vi "Empty Position.vi"(4 "Col":i32, 6 "Row":i32, 10 "Team In":i32[][](array[numeric]), 11 "Squares In":refnum<class "Square.lvclass">[][](array[class])) -> (2 "Team":i32[][](array[numeric]), 3 "Squares":refnum<class "Square.lvclass">[][](array[class]))   [LabVIEW 2020, in "SquareBattle.lvlib" / "Map.lvclass"]
uses:
  Map.lvclass
  Square/Square.lvclass
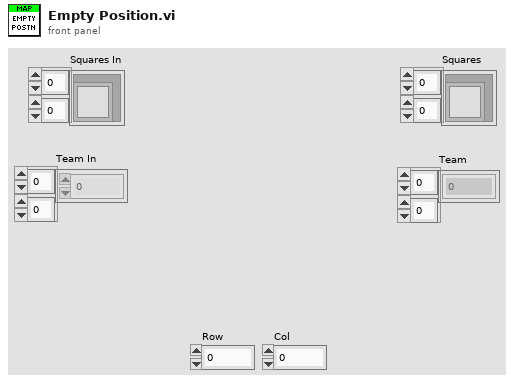
[diagram p1: front panel]
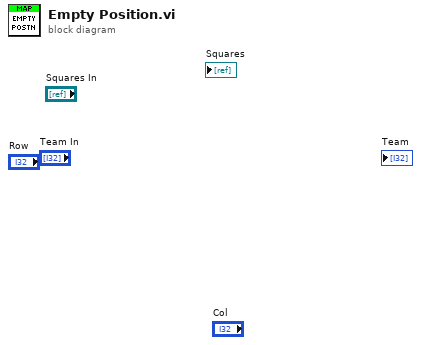
[diagram p0: block diagram]
diagram:
